vi "Write Time Stamp.vi"(8 "error in":errorcluster, 9 "user tag":i32, 10 "time stamp":timestamp, 11 "Has Timestamp in":refnum<class "Has Time Stamp.lvclass">) -> (0 "error out":errorcluster, 3 "Has Timestamp out":refnum<class "Has Time Stamp.lvclass">)   [LabVIEW 2020, in "PV Access.lvlib" / "PV Data.lvlib" / "Has Time Stamp.lvclass"]
doc: "Leave <B>time stamp</B> unwired to set the time stamp to the current time."
uses:
  Has Time Stamp.lvclass
  PV Data.lvlib
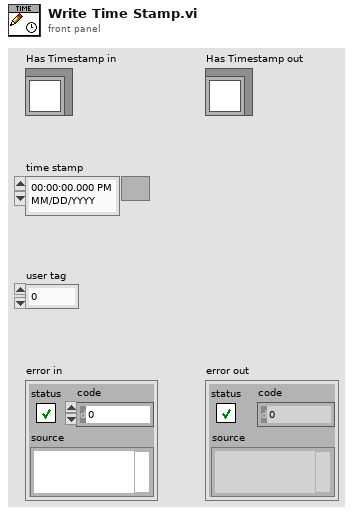
[diagram p1: front panel]
types:
  T1 = typedef "PV Access.lvlib/PV Data.lvlib/EPICS Timestamp.ctl" = cluster{"secondsPastEpoch":i64, "nanoseconds":i32, "userTag":i32}
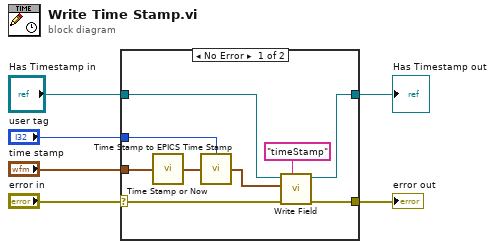
[diagram p0: block diagram]
diagram:
  n1 = case shown="No Error" "error in" {
    selector: "error in" -> [w15 w16]
    tunnel: [w14 w17] -> w5
    tunnel: [w11 w16] -> w4
    tunnel: "Has Timestamp in" -> [w10 w17]
    tunnel: "user tag" -> [w9 _]
    tunnel: "time stamp" -> [w7 _]
    frame No Error {
      n2 = call "Time Stamp or Now.vi"("time stamp in"=w7) -> ("time stamp out"=w8:timestamp)
      n3 = call "Time Stamp to EPICS Time Stamp.vi"("time stamp"=w8, "user tag"=w9) -> ("EPICS time stamp"=w12:T1)
      n4 = call-dynamic "Write Field.vi"("field"="timeStamp" ("element name"), "error in (no error)"=w15, "value"=w12, "Base Interface in"=w10) -> ("error out"=w11:errorcluster, "Base Interface out"=w14:refnum<class "Has Time Stamp.lvclass">)  [unwired: 6 in]
    }
    frame Error {
    }
  }
  "error out" <- w4
  "Has Timestamp out" <- w5
